vi "Configure Preset Level.vi"(8 "error in (no error)":errorcluster, 10 "Preset Level (5: User)":i32(ring)=5 items=["CMOS 5.0V", "CMOS 3.3V", "CMOS 2.5V", "ECL", "TTL", "User"], 11 "VISA resource name":refnum<visa-resource-name>) -> (0 "error out":errorcluster, 3 "VISA resource name out":refnum<visa-resource-name>)   [LabVIEW 2016, in "Tektronix DPO MSO 2000 4000 Series.lvlib"]
doc: "Configures the Arbitrary Function Generator preset levels to values that correspond to the logic standard specified by the argument.\n\n<B>Notes:</B>\n(1) This VI is available for MDO3000 Series only.\n\n(2) Requires the MDO3AFG option to be installed."
uses:
  Tektronix DPO MSO 2000 4000 Series.lvlib
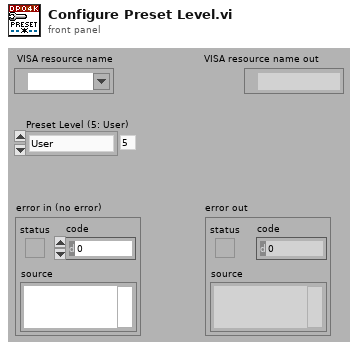
[diagram p1: front panel]
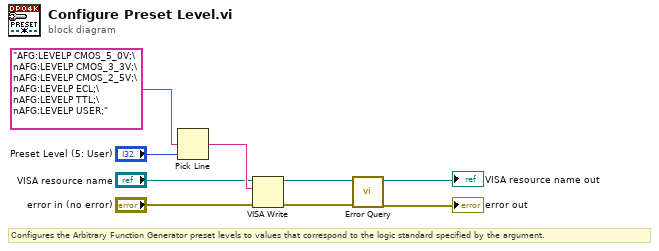
[diagram p0: block diagram]
diagram:
  # "Configures the Arbitrary Function Generator preset levels to values that correspond to the logic standard specified by the argument."
  n1 = Pick Line(multi-line string="AFG:LEVELP CMOS_5_0V;\nAFG:LEVELP CMOS_3_3V;\nAFG:LEVELP CMOS_2_5V;\nAFG:LEVELP ECL;\nAFG:LEVELP TTL;\nAFG:LEVELP USER;", line index="Preset Level (5: User)") -> (output string=w7:string)  [unwired: 1 in]
  n2 = VISA Write(VISA resource name="VISA resource name", write buffer=w7, error in (no error)="error in (no error)") -> (VISA resource name out=w5:refnum<visa-resource-name>, error out=w4:errorcluster)  [unwired: 1 out]
  n3 = call "Error Query.vi"("error in (no error)"=w4, "VISA resource name"=w5) -> ("error out"=→"error out":errorcluster, "VISA resource name out"=→"VISA resource name out":refnum<visa-resource-name>)  [unwired: 6 in, 2 out]
